vi "Main - Modules Discovery.vi"(8 "Error In":errorcluster, 11 "Allow Simulated Device? (F)":bool) -> (0 "Error Out":errorcluster, 3 "Modules Info Array":T1[](array[typedef]))   [LabVIEW 2020]
uses:
  Control/Modules Info.ctl
  <resource>/objmgr/daqmx.rc
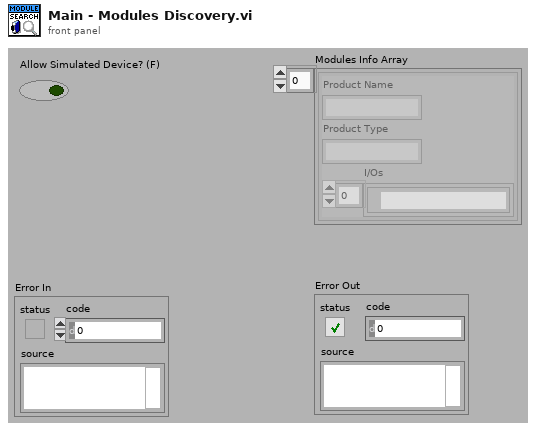
[diagram p1: front panel]
types:
  T1 = typedef "Modules Info.ctl" = cluster{"Product Name":string, "Product Type ":string, "I/Os":tag[]}
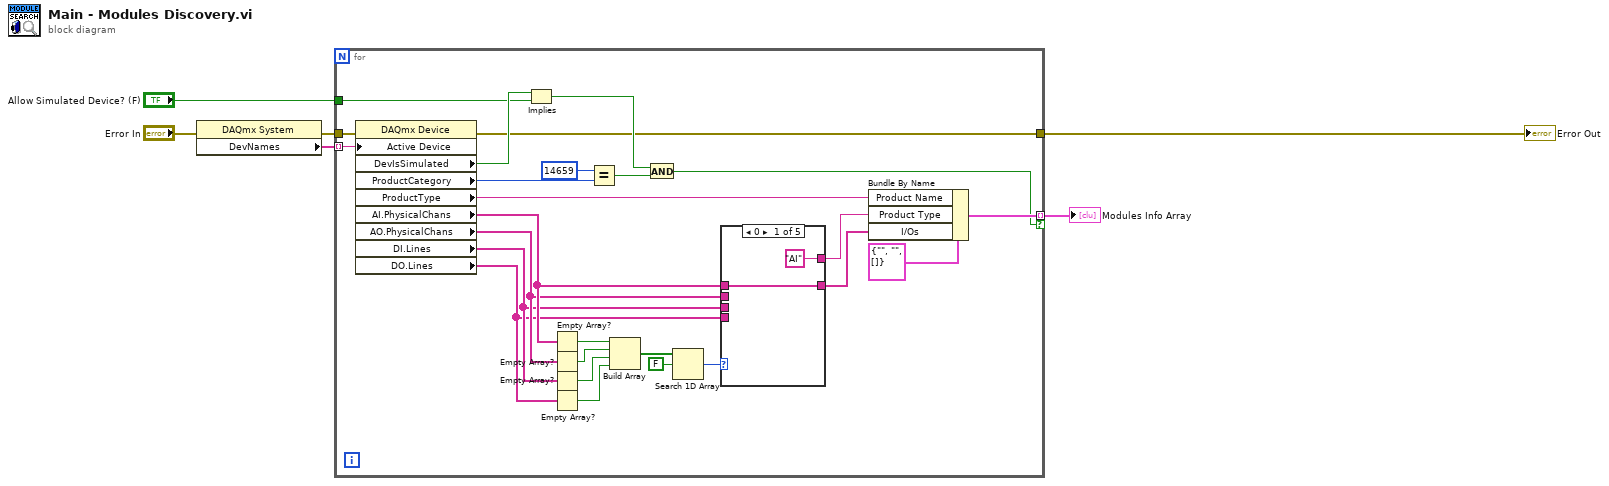
[diagram p0: block diagram]
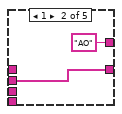
[diagram p2: hidden frame]
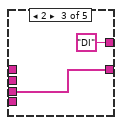
[diagram p3: hidden frame]
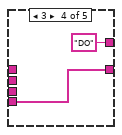
[diagram p4: hidden frame]
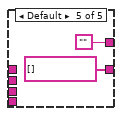
[diagram p5: hidden frame]
diagram:
  n1 = property class="DAQmx System"(error in="Error In") -> (error out=w5:errorcluster, "DevNames"=w6:tag[])  [unwired: 1 in, 1 out]
  n2 = for {
    tunnel: w6 -> [w30] mode=indexing
    tunnel: w5 -> [w29]
    tunnel: "Allow Simulated Device? (F)" -> [w20]
    tunnel: [w9] -> w1 mode=indexing if=w8
    tunnel: [w7] -> w2
    n3 = property class="DAQmx Device"(error in=w29, "Active Device"=w30) -> (error out=w7:errorcluster, "DevIsSimulated"=w21:bool, "ProductCategory"=w32:i32, "ProductType"=w12:string, "AI.PhysicalChans"=w17:tag[], "AO.PhysicalChans"=w16:tag[], "DI.Lines"=w15:tag[], "DO.Lines"=w14:tag[])  [unwired: 1 in, 1 out]
    n4 = Implies(1:w20, 2:w21) -> (0:w22:bool)
    n5 = Empty Array?(array=w17) -> (empty?=w28:bool)
    n6 = Empty Array?(array=w16) -> (empty?=w27:bool)
    n7 = Empty Array?(array=w15) -> (empty?=w26:bool)
    n8 = Empty Array?(array=w14) -> (empty?=w25:bool)
    n9 = Equal?(x=14659 ("y"), y=w32) -> (x = y?=w19:bool)
    n10 = Build Array(w28, w27, w26, w25) -> (w24:bool[])
    n11 = And(x=w22, y=w19) -> (x .and. y?=w8:bool)
    n12 = Search 1D Array(1D array=w24, element=FALSE) -> (index of element=w18:i32)  [unwired: 1 in]
    n13 = case shown="0" w18 {
      tunnel: w17 -> [w34 _ _ _ _]
      tunnel: w16 -> [_ w36 _ _ _]
      tunnel: w15 -> [_ _ w37 _ _]
      tunnel: w14 -> [_ _ _ w39 _]
      tunnel: [w34 w36 w37 w39 tag[] [] ("DO.Lines")] -> w10
      tunnel: ["AI" "AO" "DI" "DO" ""] -> w11
      frame 0 {
      }
      frame 1 {
      }
      frame 2 {
      }
      frame 3 {
      }
      frame Default {
      }
    }
    n14 = Bundle By Name(cluster=T1 {"Product Name"="", "Product Type "="", "I/Os"=[]} ("Modules Info"), "Product Name"=w12, "Product Type"=w11, "I/Os"=w10) -> (w9:T1)
  }
  "Modules Info Array" <- w1
  "Error Out" <- w2
